vi "ChangeWebBrowserBehaviour.vi"(8 "error in (no error)":errorcluster, 11 "object in":refnum<class "WebBrowser_Mgmt.lvclass">) -> (0 "error out":errorcluster, 3 "object out":refnum<class "WebBrowser_Mgmt.lvclass">)   [LabVIEW 2016, in "WebBrowser_Mgmt.lvclass"]
uses:
  WebBrowser_Mgmt.lvclass
  WebBrowser_Mgmt.lvclass/WebBrowser_Mgmt.ctl
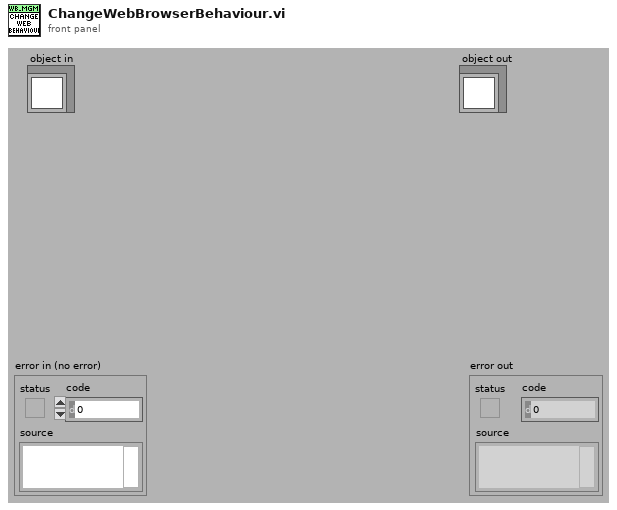
[diagram p1: front panel]
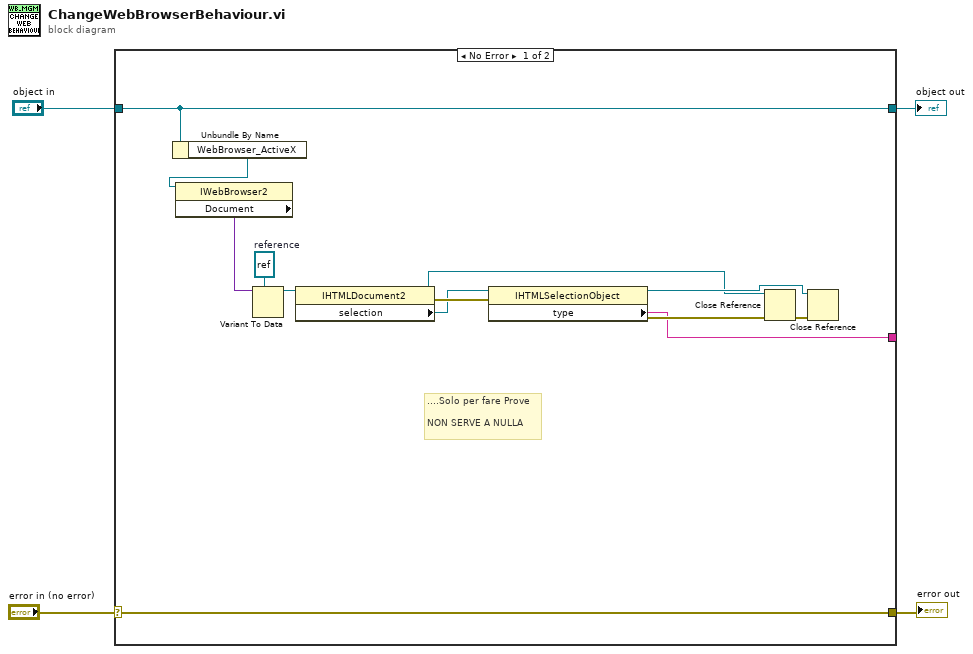
[diagram p0: block diagram]
diagram:
  n1 = case shown="No Error" "error in (no error)" {
    selector: "error in (no error)" -> [w17 w19]
    tunnel: [w17 w19] -> w3
    tunnel: [w16 w18] -> w1
    tunnel: "object in" -> [w16 w18]
    tunnel: [w10 _] -> _
    frame No Error {
      w8 = refnum<k7> refnum  # reference
      # "....Solo per fare Prove\n\nNON SERVE A NULLA"
      n2 = Unbundle By Name(w16) -> ("WebBrowser_ActiveX"=w9:refnum<k7>)
      n3 = property class="IWebBrowser2"(reference=w9) -> ("Document"=w15:variant)  [unwired: 1 in, 2 out]
      n4 = Variant To Data(type=w8, Variant=w15) -> (data=w5:refnum<k7>)  [unwired: 1 in, 1 out]
      n5 = property class="IHTMLDocument2"(reference=w5) -> (reference out=w7:refnum<k7>, error out=w14:errorcluster, "selection"=w6:refnum<k7>)  [unwired: 1 in]
      n6 = property class="IHTMLSelectionObject"(reference=w6, error in=w14) -> (reference out=w12:refnum<k7>, error out=w11:errorcluster, "type"=w10:string)
      n7 = Close Reference(reference=w7, error in (no error)=w11) -> (error out=w13:errorcluster)
      n8 = Close Reference(reference=w12, error in (no error)=w13) -> ()  [unwired: 1 out]
    }
    frame Error {
    }
  }
  "error out" <- w3
  "object out" <- w1
